vi "Push.vi"(10 "Element":T1, 11 "POTTypedCircularBuffer in":refnum<class "ErrorLogBuffer.lvclass">) -> (3 "POTTypedCircularBuffer out":refnum<class "ErrorLogBuffer.lvclass">)   [LabVIEW 2024, in "ErrorLogBuffer.lvclass"]
uses:
  ErrorLogBuffer.lvclass
  Type.ctl
  RQMHCore/ErrorReporting/Record/LogRecord.lvclass
  ErrorLogBuffer.lvclass/ErrorLogBuffer.ctl
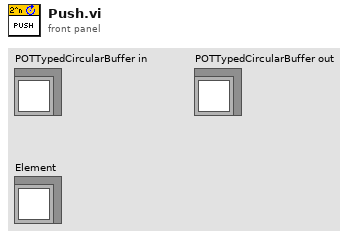
[diagram p1: front panel]
types:
  T1 = typedef "ErrorLogBuffer.lvclass/Type.ctl" = refnum<class "LogRecord.lvclass">
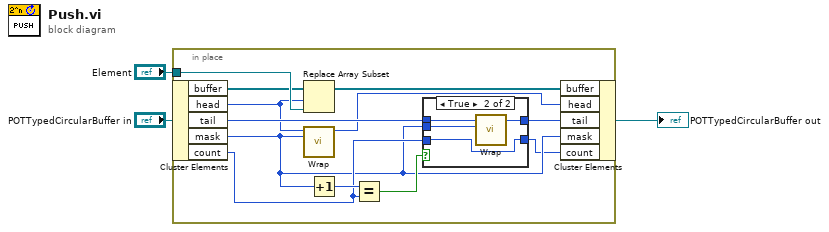
[diagram p0: block diagram]
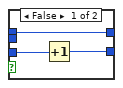
[diagram p2: hidden frame]
diagram:
  n1 = in-place {
    in-place-border: "Element" -> [w14]
    n2 = in-place-cluster #1("POTTypedCircularBuffer in") -> ("buffer"=w10:T1[], "head"=w9:i32, "tail"=w13:i32, "mask"=w5:i32, "count"=w6:i32)
    n3 = Replace Array Subset(array=w10, new element=w14, index=w9) -> (w15:T1[])
    n4 = call "Wrap.vi"("mask"=w5, "index"=w9) -> ("wrapped"=w11:i32)  [unwired: 9 in]
    n5 = Increment(x=w5) -> (x+1=w8:i32)
    n6 = Equal?(x=w8, y=w6) -> (x = y?=w7:bool)
    n7 = case shown="True" w7 {
      tunnel: w13 -> [w18 w22]
      tunnel: w5 -> [_ w21]
      tunnel: [w18 w20] -> w12
      tunnel: w6 -> [w17 w19]
      tunnel: [w16 w19] -> w4
      frame False {
        n8 = Increment(x=w17) -> (x+1=w16:i32)
      }
      frame True {
        n9 = call "Wrap.vi"("mask"=w21, "index"=w22) -> ("wrapped"=w20:i32)  [unwired: 9 in]
      }
    }
    n10 = in-place-cluster #1("buffer"=w15, "head"=w11, "tail"=w12, "mask"=w5, "count"=w4) -> (→"POTTypedCircularBuffer out":refnum<class "ErrorLogBuffer.lvclass">)
  }
